vi "PCO_Single_Signal_Desc.vi"() -> (0 "PCO_Single_Signal_Desc":T2, 1 "PCO_Single_Signal_Desc_Raw":T1, 2 "Length":u16, 3 "Raw_Length":u16)   [LabVIEW 2019, in "SDK.lvlib" / "Structures.lvlib"]
doc: "Use this template to build a VI to use as a subVI."
uses:
  Structures.lvlib
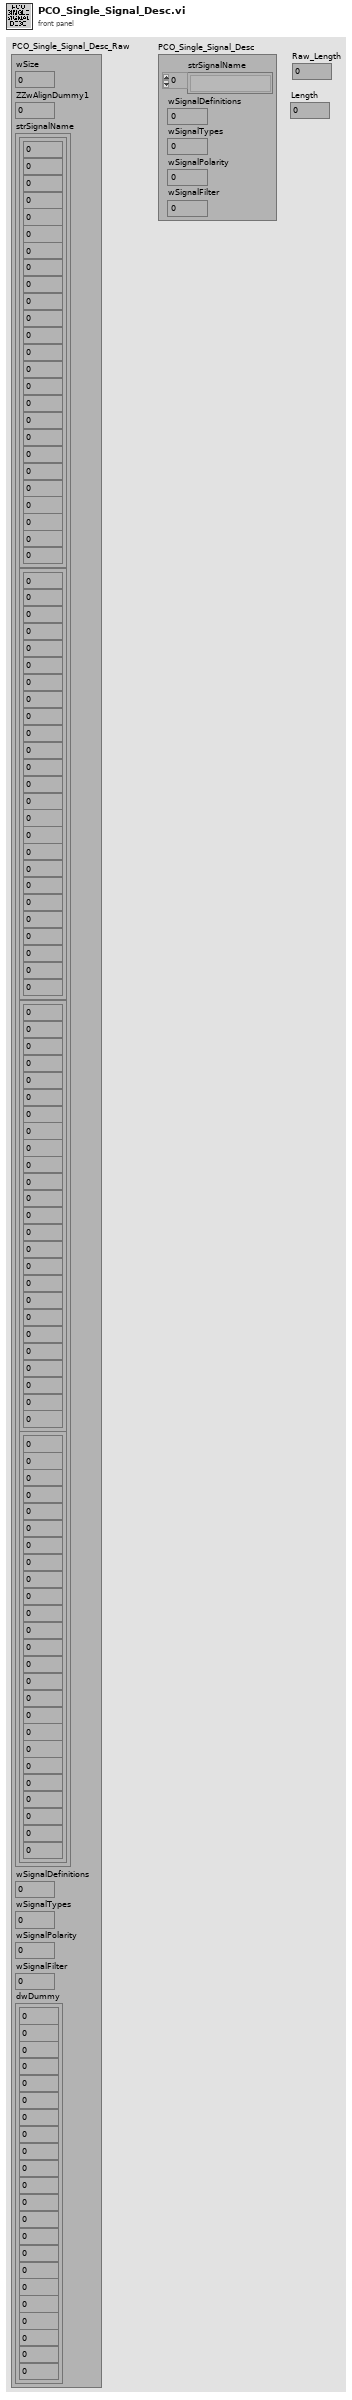
[diagram p1: front panel]
types:
  T1 = cluster{"wSize":u16, "ZZwAlignDummy1":u16, "strSignalName":cluster{cluster{u8, u8, u8, u8, u8, u8, u8, u8, u8, u8, u8, u8, u8, u8, u8, u8, u8, u8, u8, u8, u8, u8, u8, u8, u8}, cluster{u8, u8, u8, u8, u8, u8, u8, u8, u8, u8, u8, u8, u8, u8, u8, u8, u8, u8, u8, u8, u8, u8, u8, u8, u8}, cluster{u8, u8, u8, u8, u8, u8, u8, u8, u8, u8, u8, u8, u8, u8, u8, u8, u8, u8, u8, u8, u8, u8, u8, u8, u8}, cluster{u8, u8, u8, u8, u8, u8, u8, u8, u8, u8, u8, u8, u8, u8, u8, u8, u8, u8, u8, u8, u8, u8, u8, u8, u8}}, "wSignalDefinitions":u16, "wSignalTypes":u16, "wSignalPolarity":u16, "wSignalFilter":u16, "dwDummy":cluster{u32, u32, u32, u32, u32, u32, u32, u32, u32, u32, u32, u32, u32, u32, u32, u32, u32, u32, u32, u32, u32, u32}}
  T2 = cluster{"strSignalName":string[], "wSignalDefinitions":u16, "wSignalTypes":u16, "wSignalPolarity":u16, "wSignalFilter":u16}
  T3 = cluster{u32, u32, u32, u32, u32, u32, u32, u32, u32, u32, u32, u32, u32, u32, u32, u32, u32, u32, u32, u32, u32, u32}
  T4 = cluster{cluster{u8, u8, u8, u8, u8, u8, u8, u8, u8, u8, u8, u8, u8, u8, u8, u8, u8, u8, u8, u8, u8, u8, u8, u8, u8}, cluster{u8, u8, u8, u8, u8, u8, u8, u8, u8, u8, u8, u8, u8, u8, u8, u8, u8, u8, u8, u8, u8, u8, u8, u8, u8}, cluster{u8, u8, u8, u8, u8, u8, u8, u8, u8, u8, u8, u8, u8, u8, u8, u8, u8, u8, u8, u8, u8, u8, u8, u8, u8}, cluster{u8, u8, u8, u8, u8, u8, u8, u8, u8, u8, u8, u8, u8, u8, u8, u8, u8, u8, u8, u8, u8, u8, u8, u8, u8}}
  T5 = cluster{string[], "wSignalDefinitions":u16, "wSignalTypes":u16, "wSignalPolarity":u16, "wSignalFilter":u16}
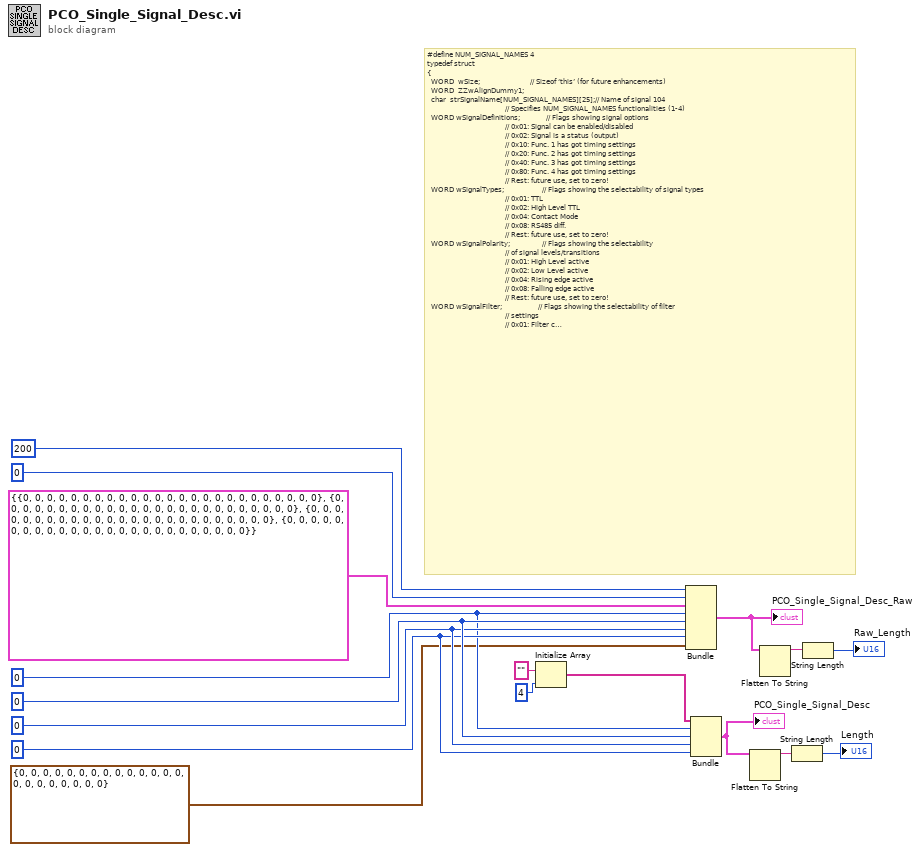
[diagram p0: block diagram]
diagram:
  w6 = u16 0 ("wSignalDefinitions")
  w8 = u16 0 ("wSignalFilter")
  w9 = u16 0 ("wSignalPolarity")
  w10 = u16 0 ("wSignalTypes")
  # "#define NUM_SIGNAL_NAMES 4\ntypedef struct\n{\n  WORD  wSize;                         // Sizeof ‘this’ (for future enhancements)\n  WORD  ZZwAlignDummy1;\n  char  strSignalName[NUM_SIGNAL_NAMES][25];// Name of signal 104\n                                       // Specifies NUM_SIGNAL_NAMES functionalities (1-4)\n  WORD wSignalDefinitions;             // Flags showing signal options\n                                       // 0x01: Signal can be enabled/disabled\n                                       // 0x02: Signal is a status (output)\n                                       // 0x10: Func. 1 has got timing settings\n                                       // 0x20: Func. 2 has got timing settings\n                                       // 0x40: Func. 3 has got timing settings\n                                       // 0x80: Func. 4 has got timing settings\n                                       // Rest: future use, set to zero!\n  WORD wSignalTypes;                   // Flags showing the selectability of signal types\n                                       // 0x01: TTL\n                                       // 0x02: High Level TTL\n                                       // 0x04: Contact Mode\n                                       // 0x08: RS485 diff.\n                                       // Rest: future use, set to zero!\n  WORD wSignalPolarity;                // Flags showing the selectability\n                                       // of signal levels/transitions\n                                       // 0x01: High Level active\n                                       // 0x02: Low Level active\n                                       // 0x04: Rising edge active\n                                       // 0x08: Falling edge active\n                                       // Rest: future use, set to zero!\n  WORD wSignalFilter;                  // Flags showing the selectability of filter\n                                       // settings\n                                       // 0x01: Filter can be switched off (t > ~65ns)\n                                       // 0x02: Filter can be switched to medium (t > ~1us)\n                                       // 0x04: Filter can be switched to high (t > ~100ms) 112\n  DWORD dwDummy[22];                   // reserved for future use. (only in SDK) 200\n}PCO_Single_Signal_Desc;"
  n1 = Initialize Array("", 4 ("dimension size")) -> (w1:string[])
  n2 = Bundle("wSize"=u16 200, "ZZwAlignDummy1"=u16 0, "strSignalName"=T4 {{0, 0, 0, 0, 0, 0, 0, 0, 0, 0, 0, 0, 0, 0, 0, 0, 0, 0, 0, 0, 0, 0, 0, 0, 0}, {0, 0, 0, 0, 0, 0, 0, 0, 0, 0, 0, 0, 0, 0, 0, 0, 0, 0, 0, 0, 0, 0, 0, 0, 0}, {0, 0, 0, 0, 0, 0, 0, 0, 0, 0, 0, 0, 0, 0, 0, 0, 0, 0, 0, 0, 0, 0, 0, 0, 0}, {0, 0, 0, 0, 0, 0, 0, 0, 0, 0, 0, 0, 0, 0, 0, 0, 0, 0, 0, 0, 0, 0, 0, 0, 0}}, "wSignalDefinitions"=w6, "wSignalTypes"=w10, "wSignalPolarity"=w9, "wSignalFilter"=w8, "dwDummy"=T3 {0, 0, 0, 0, 0, 0, 0, 0, 0, 0, 0, 0, 0, 0, 0, 0, 0, 0, 0, 0, 0, 0}) -> (w7:T1)  [unwired: 1 in]
  "PCO_Single_Signal_Desc_Raw" <- w7
  n3 = Bundle(w1, "wSignalDefinitions"=w6, "wSignalTypes"=w10, "wSignalPolarity"=w9, "wSignalFilter"=w8) -> (w17:T5)  [unwired: 1 in]
  "PCO_Single_Signal_Desc" <- w17
  n4 = Flatten To String(anything=w17) -> (data string=w16:string)  [unwired: 3 in, 2 out]
  n5 = Flatten To String(anything=w7) -> (data string=w15:string)  [unwired: 3 in, 2 out]
  n6 = String Length(string=w16) -> (length=→"Length":i32)
  n7 = String Length(string=w15) -> (length=→"Raw_Length":i32)
